vi "Read Val.vi"(8 "error in (no error)":errorcluster, 11 "Update Switch MSG in":refnum<class "Update Switch MSG.lvclass">) -> (0 "error out":errorcluster, 2 "Val":bool, 3 "Update Switch MSG out":refnum<class "Update Switch MSG.lvclass">)   [LabVIEW 2014, in "Update Switch MSG.lvclass"]
uses:
  Update Switch MSG.lvclass
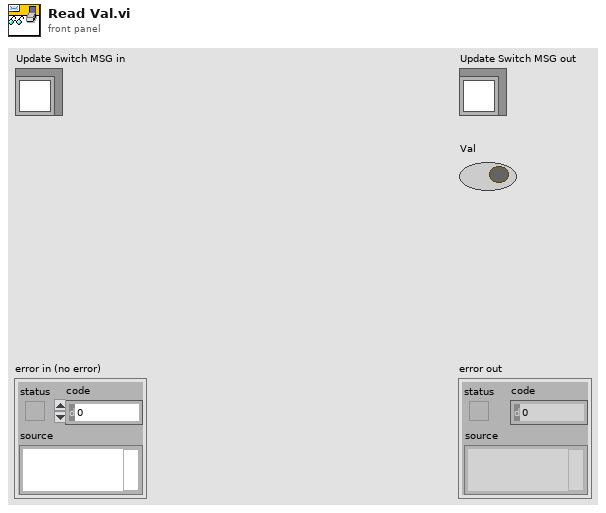
[diagram p1: front panel]
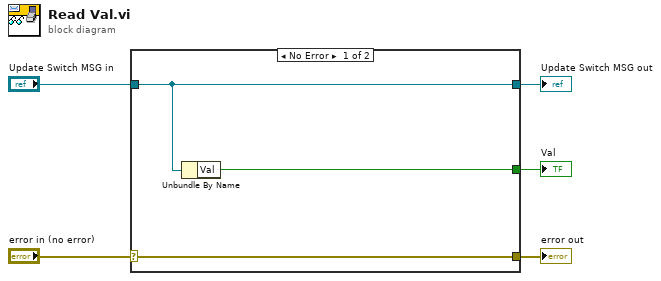
[diagram p0: block diagram]
diagram:
  n1 = case shown="No Error" "error in (no error)" {
    selector: "error in (no error)" -> [w8 w9]
    tunnel: [w8 w9] -> w4
    tunnel: [w7 w10] -> w2
    tunnel: "Update Switch MSG in" -> [w7 w10]
    tunnel: [w6 _] -> w1
    frame No Error {
      n2 = Unbundle By Name(w7) -> ("Val"=w6:bool)
    }
    frame Error {
    }
  }
  "error out" <- w4
  "Update Switch MSG out" <- w2
  "Val" <- w1
